vi "reset locks.vi"(8 "error in (no error)":errorcluster) -> (0 "error out":errorcluster, 3 "function return":i32)   [LabVIEW 2012, in "libximc.lvlib"]
doc: "result_t XIMC_API reset_locks ();"
uses:
  libximc.lvlib
  libximc.dll
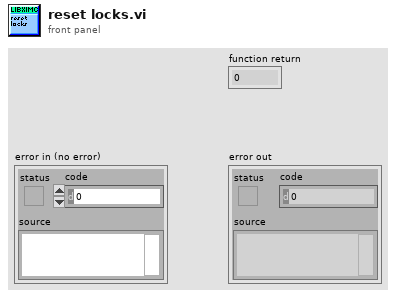
[diagram p1: front panel]
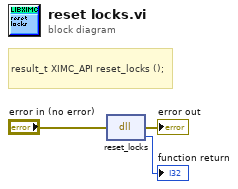
[diagram p0: block diagram]
diagram:
  # "result_t XIMC_API reset_locks ();"
  n1 = dll-call lib="E:/labview-2.12.1-Labview_12.0/ximcLVx32/libximc.*" fn="reset_locks"(error in="error in (no error)") -> (error out=→"error out":errorcluster, →"function return":i32)  [unwired: 2 in, 1 out]
